vi "2.vi"(7 "Kezelõpult":T1={"Filt_alsó"=750.0, "Filt_felsõ"=7400.0, "Optikai elem hossza (km)"=0.000445, "Referencia hullámhossz (nm)"=800.0, " Illesztendõ polinom fokszáma"=7, "Megjegyzések"=""}, 8 "error in (no error)":errorcluster, 11 "adat":T2) -> (0 "error out":errorcluster, 2 "Waveform Graph 2":dbl[][](graph), 3 "adat":T2)   [LabVIEW 2016]
doc: "0-val való feltöltés, iDFFT, filterezés, DFFT."
uses:
  adat.ctl
  <vilib>/Analysis/2dsp.llb/Inverse Complex FFT.vi
  <vilib>/Analysis/2dsp.llb/Complex FFT.vi
  <vilib>/Analysis/NI_AALPro.lvlib
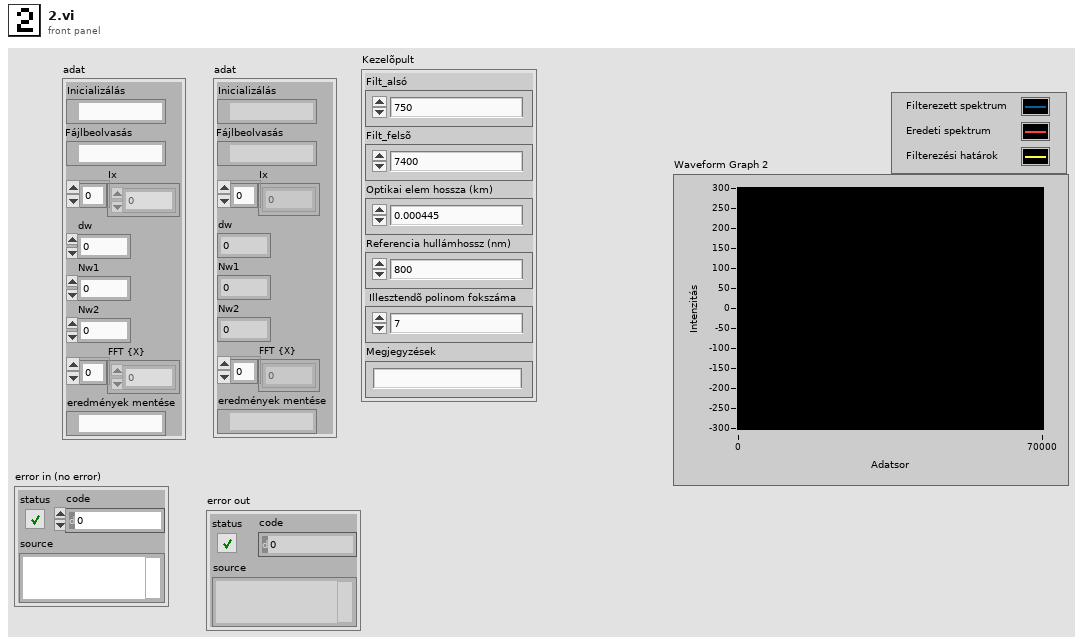
[diagram p1: front panel]
types:
  T1 = typedef "kezelõpult.ctl" = cluster{"Filt_alsó":dbl, "Filt_felsõ":dbl, "Optikai elem hossza (km)":dbl, "Referencia hullámhossz (nm)":dbl, " Illesztendõ polinom fokszáma":i32, "Megjegyzések":string}
  T2 = typedef "adat.ctl" = cluster{"Inicializálás":path, "Fájlbeolvasás":path, "Ix":dbl[], "dw":dbl, "Nw1":dbl, "Nw2":dbl, "FFT {X}":cdb[], "eredmények mentése":path}
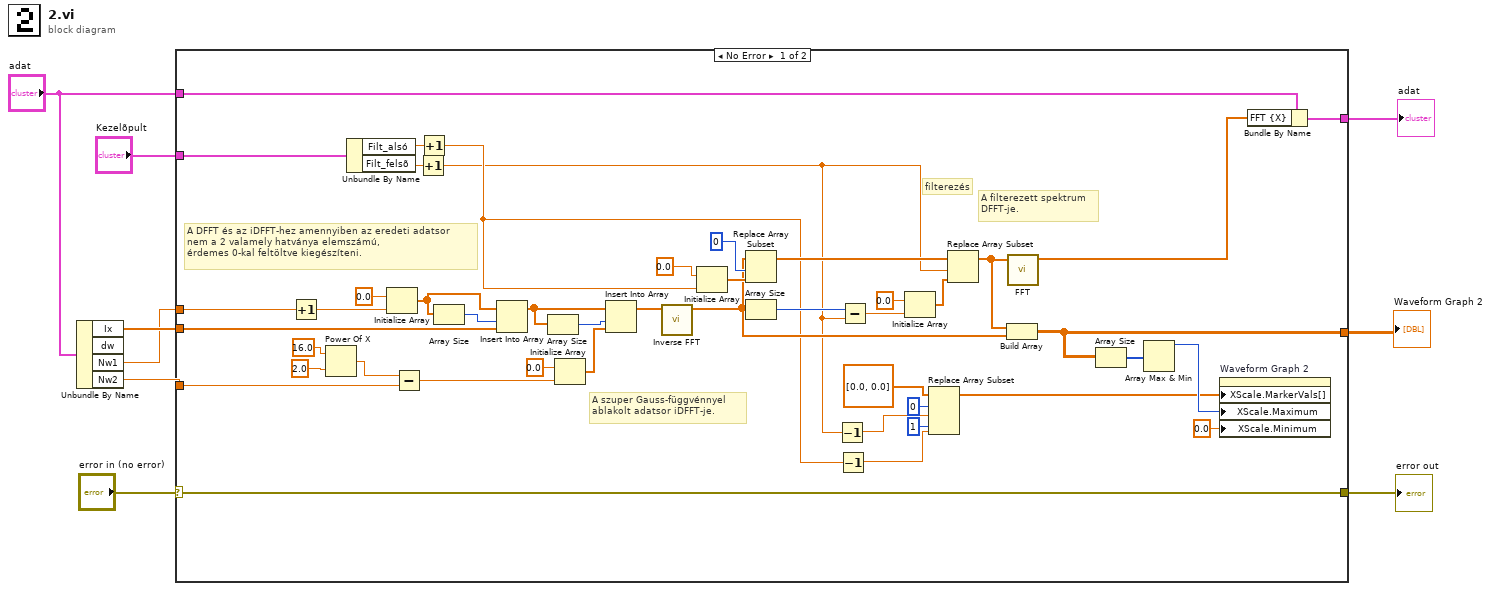
[diagram p0: block diagram]
diagram:
  n1 = Unbundle By Name("adat") -> ("Ix"=w5:dbl[], "Nw1"=w4:dbl, "Nw2"=w6:dbl)  [unwired: 1 out]
  n2 = case shown="No Error" "error in (no error)" {
    selector: "error in (no error)" -> [w14 w56]
    tunnel: w6 -> [w42 _]
    tunnel: w5 -> [w39 _]
    tunnel: w4 -> [w36 _]
    tunnel: [w28 _] -> w9
    tunnel: "Kezelõpult" -> [w10 _]
    tunnel: [w14 w56] -> w7
    tunnel: "adat" -> [w13 w55]
    tunnel: [w11 w55] -> w2
    frame No Error {
      # "A filterezett spektrum \nDFFT-je."
      # "filterezés"
      # "A DFFT és az iDFFT-hez amennyiben az eredeti adatsor \nnem a 2 valamely hatványa elemszámú,\nérdemes 0-kal feltöltve kiegészíteni."
      # "A szuper Gauss-függvénnyel \nablakolt adatsor iDFFT-je."
      n3 = Increment(x=w36) -> (x+1=w32:dbl)
      n4 = Power Of X(1:2.0 ("x"), 2:16.0 ("y")) -> (0:w41:dbl)
      n5 = Unbundle By Name(w10) -> ("Filt_alsó"=w18:dbl, "Filt_felsõ"=w17:dbl)
      n6 = Initialize Array(0.0, w32) -> (w38:dbl[])
      n7 = Subtract(x=w41, y=w42) -> (x-y=w31:dbl)
      n8 = Increment(x=w17) -> (x+1=w15:dbl)
      n9 = Increment(x=w18) -> (x+1=w16:dbl)
      n10 = Array Size(array=w38) -> (size(s)=w37:i32)
      n11 = Insert Into Array(array=w38, index=w37, new element=w39) -> (w45:dbl[])
      n12 = Array Size(array=w45) -> (size(s)=w44:i32)
      n13 = Initialize Array(0.0, w31) -> (w43:dbl[])
      n14 = Insert Into Array(array=w45, index=w44, new element=w43) -> (w46:dbl[])
      n15 = call-poly <vilib>:"Inverse FFT.vi"("FFT {X}"=w46) -> ("X"=w29:cdb[])  [unwired: 9 in, 1 out]
      n16 = Initialize Array(0.0, w16) -> (w48:dbl[])
      n17 = Replace Array Subset(array=w29, new element=w48, index=0) -> (w54:cdb[])
      n18 = Array Size(array=w29) -> (size(s)=w51:i32)
      n19 = Decrement(x=w15) -> (x-1=w23:dbl)
      n20 = Decrement(x=w16) -> (x-1=w20:dbl)
      n21 = Subtract(x=w51, y=w15) -> (x-y=w52:dbl)
      n22 = Initialize Array(0.0, w52) -> (w53:dbl[])
      n23 = Replace Array Subset(array=dbl[] [0.0, 0.0], new element #1=w23, index #1=0 ("index"), new element #2=w20, index #2=1 ("index")) -> (w19:dbl[])
      n24 = Replace Array Subset(array=w54, new element=w53, index=w15) -> (w30:cdb[])
      n25 = Build Array(w30, w29) -> (w28:cdb[][])
      n26 = call-poly <vilib>:"FFT.vi"("X"=w30) -> ("FFT {X}"=w12:cdb[])  [unwired: 9 in, 1 out]
      n27 = Array Size(array=w28) -> (size(s)=w25:i32[])
      n28 = Array Max & Min(array=w25) -> (max value=w27:i32)  [unwired: 3 out]
      n29 = property on="Waveform Graph 2" class="WFGraph (strict)"("XScale.MarkerVals[]"=w19, "XScale.Maximum"=w27, "XScale.Minimum"=0.0 ("X Scale.Range:Minimum")) -> ()  [unwired: 2 in, 2 out]
      n30 = Bundle By Name(cluster=w13, "FFT {X}"=w12) -> (w11:T2)
    }
    frame Error {
    }
  }
  "Waveform Graph 2" <- w9
  "error out" <- w7
  "adat" <- w2
